vi "Button_handling1.vi"(7 "connect":bool, 10 "Z_Source":T2=enum."local disabled", 11 "Z_HSwitch":bool) -> (1 "Z_HSwitch_out":T1, 2 "Z1 ind":u8(ring), 3 "Write Enable":bool)   [LabVIEW 2019]
uses:
  Y_source.ctl
  Button state1.ctl
  Trigers/D^.vi
  Logik/fronts.vi
  Timer Delay/Timers.lvlib
  Counter/Counter.lvlib
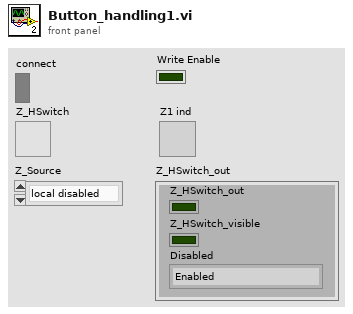
[diagram p1: front panel]
types:
  T1 = cluster{"Z_HSwitch_out":bool, "Z_HSwitch_visible":bool, "Disabled":enum8{"Enabled", "Disabled", "Disabled and Grayed Out"}}
  T2 = typedef "Y_source.ctl" = enum8{"initialize", "local disabled", "local hand", "hand", "auto", "dist"}
  T3 = enum8{"Enabled", "Disabled", "Disabled and Grayed Out"}
  T4 = typedef "Button state1.ctl" = enum16{"set init", "init", "set not connect", "not connect", "set local disabled", "local disabled", "set local hand", "local hand", "set hand", "hand", "set auto", "auto", "set dist", "dist"}
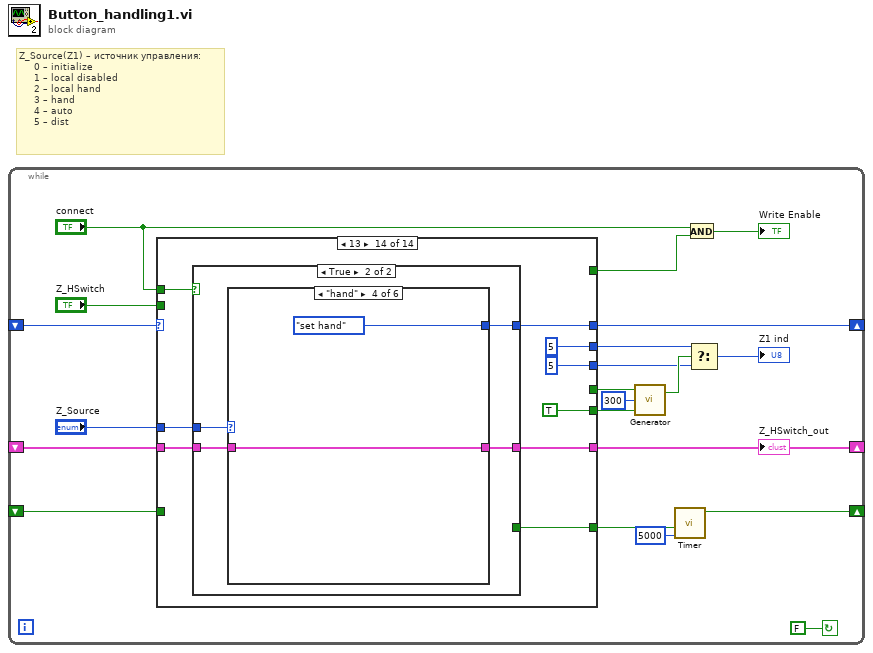
[diagram p0: block diagram]
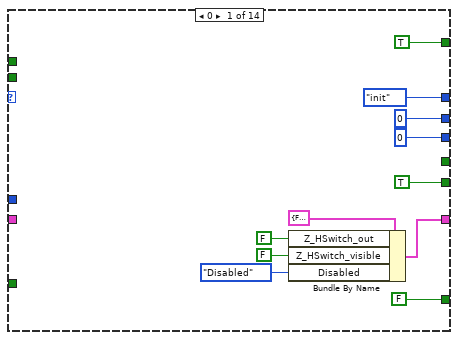
[diagram p2: hidden frame]
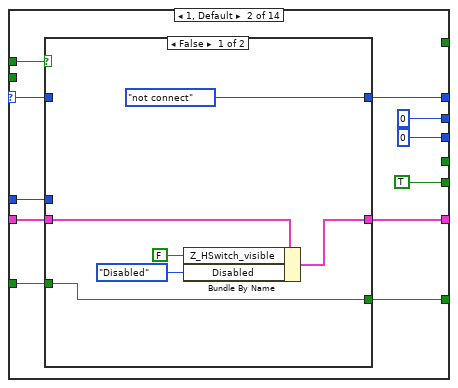
[diagram p3: hidden frame]
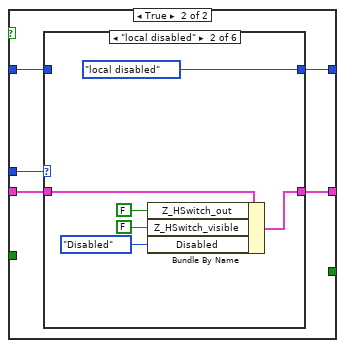
[diagram p4: hidden frame]
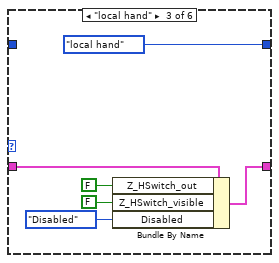
[diagram p6: hidden frame]
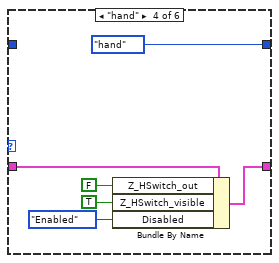
[diagram p7: hidden frame]
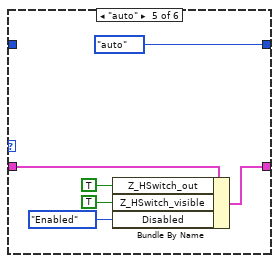
[diagram p8: hidden frame]
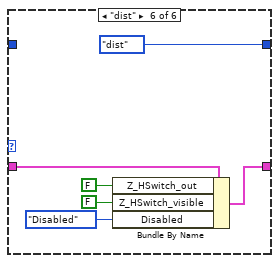
[diagram p9: hidden frame]
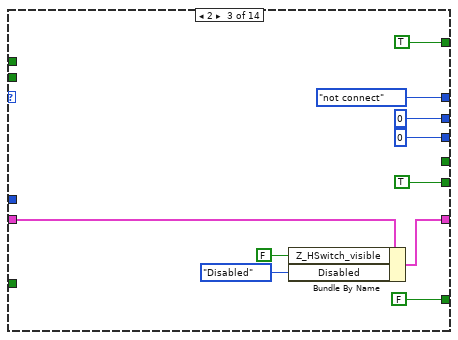
[diagram p10: hidden frame]
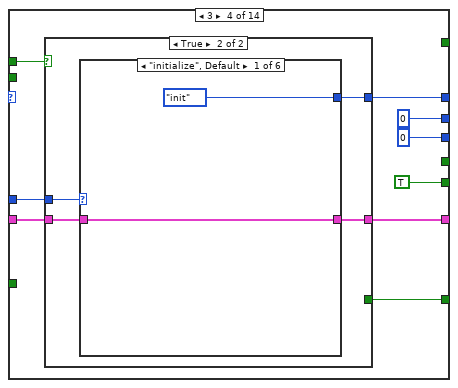
[diagram p11: hidden frame]
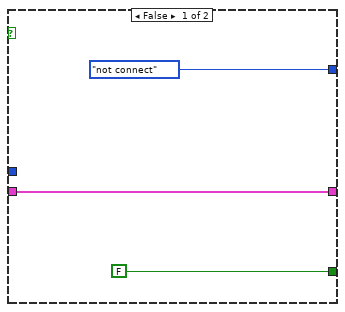
[diagram p12: hidden frame]
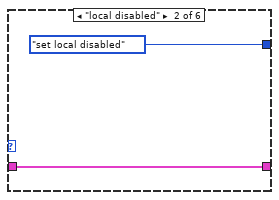
[diagram p13: hidden frame]
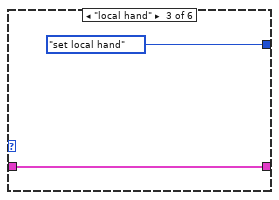
[diagram p14: hidden frame]
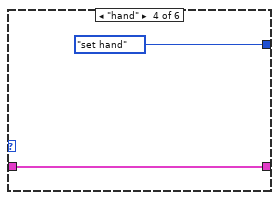
[diagram p15: hidden frame]
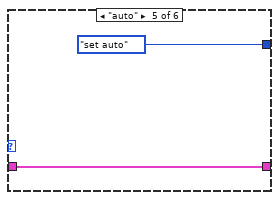
[diagram p16: hidden frame]
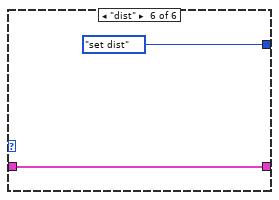
[diagram p17: hidden frame]
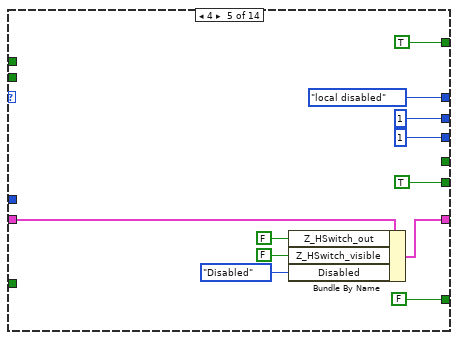
[diagram p18: hidden frame]
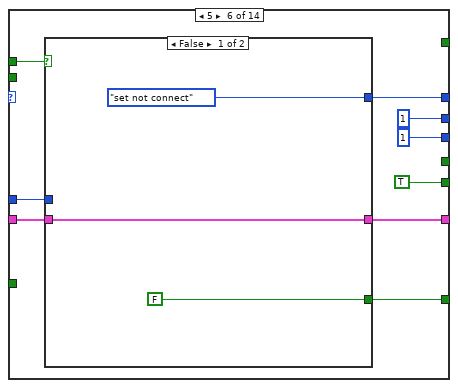
[diagram p19: hidden frame]
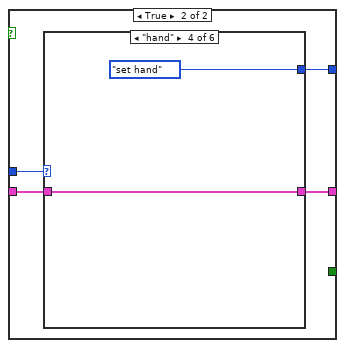
[diagram p20: hidden frame]
diagram:
  # "Z_Source(Z1) – источник управления:\n     0 – initialize\n     1 – local disabled\n     2 – local hand\n     3 – hand\n     4 – аuto\n     5 – dist"
  n1 = while {
    shift-right: [w21] -> _
    shift-left: _ -> [w7]
    shift-right: [w8] -> _
    shift-left: _ -> [w20]
    shift-right: [w4] -> _
    shift-left: _ -> [w9]
    stop <- FALSE continue-if-true
    n2 = case shown="13" w7 {
      selector: w7 -> [_ w33 _ _ _ _ _ _ _ _ _ _ _ _]
      tunnel: "connect" -> [_ w42 _ w104 _ w141 _ w180 w211 w255 w307 w351 _ w412]
      tunnel: "Z_HSwitch" -> [_ _ _ _ _ _ _ _ _ w257 _ w353 _ _]
      tunnel: [Button_state1."init" ("f 3") w43 Button_state1."not connect" ("f 3") w105 Button_state1."local disabled" ("f 3") w136 Button_state1."local hand" ("f 3") w179 w212 w256 w308 w352 Button_state1."dist" ("f 3") w413] -> w21
      tunnel: "Z_Source" -> [_ w41 _ w103 _ w138 _ w177 w210 w254 w306 w350 _ w411]
      tunnel: w20 -> [_ w34 _ _ _ _ _ _ w205 _ w301 _ _ _]
      tunnel: [FALSE ("Z_ASwitch") w40 FALSE ("Z_ASwitch") w102 FALSE ("Z_ASwitch") w137 FALSE ("Z_ASwitch") w175 w209 w253 w305 w349 FALSE ("Z_ASwitch") w408] -> w19
      tunnel: [u8 0 ("Z1 ind") u8 0 ("Z1 ind") u8 0 ("Z1 ind") u8 0 ("Z1 ind") u8 1 ("Z1 ind") u8 1 ("Z1 ind") u8 2 ("Z1 ind") u8 2 ("Z1 ind") u8 3 ("Z1 ind") u8 4 ("Z1 ind") u8 4 ("Z1 ind") u8 4 ("Z1 ind") u8 5 ("Z1 ind") u8 5 ("Z1 ind")] -> w12
      tunnel: [_ _ _ _ _ _ _ _ TRUE ("Z_ASwitch") w250 TRUE ("Z_ASwitch") w345 _ _] -> w17
      tunnel: [u8 0 ("Z1 ind") u8 0 ("Z1 ind") u8 0 ("Z1 ind") u8 0 ("Z1 ind") u8 1 ("Z1 ind") u8 1 ("Z1 ind") u8 2 ("Z1 ind") u8 2 ("Z1 ind") u8 4 ("Z1 ind") u8 3 ("Z1 ind") u8 3 ("Z1 ind") u8 4 ("Z1 ind") u8 5 ("Z1 ind") u8 5 ("Z1 ind")] -> w16
      tunnel: [TRUE ("Z_ASwitch") TRUE ("Z_ASwitch") TRUE ("Z_ASwitch") TRUE ("Z_ASwitch") TRUE ("Z_ASwitch") TRUE ("Z_ASwitch") TRUE ("Z_ASwitch") TRUE ("Z_ASwitch") _ w249 _ w346 TRUE ("Z_ASwitch") TRUE ("Z_ASwitch")] -> w15
      tunnel: [TRUE ("Z_ASwitch") _ TRUE ("Z_ASwitch") _ TRUE ("Z_ASwitch") _ TRUE ("Z_ASwitch") _ _ w246 _ w342 TRUE ("Z_ASwitch") _] -> w11
      tunnel: [w23 w36 w87 w98 w125 w140 w164 w178 w204 w248 w300 w344 w397 w409] -> w4
      tunnel: w9 -> [_ w35 w88 w97 w126 w139 w165 w176 w203 w247 w299 w343 w398 w410]
      frame 0 {
        # "local hand"
        n3 = Bundle By Name(cluster=T1 {"Z_HSwitch_out"=FALSE, "Z_HSwitch_visible"=FALSE, "Disabled"=enum."Enabled"} ("Z_HSwitch_out"), "Z_HSwitch_out"=FALSE ("Z_ASwitch"), "Z_HSwitch_visible"=FALSE ("Z_ASwitch"), "Disabled"=T3."Disabled") -> (w23:T1)
      }
      frame 1, Default {
        # "local hand"
        n4 = case shown="False" w42 {
          tunnel: [Button_state1."not connect" ("f 3") w54] -> w43
          tunnel: w41 -> [_ w53]
          tunnel: [w48 _] -> w40
          tunnel: [w44 w52] -> w36
          tunnel: w35 -> [w45 w51]
          tunnel: w34 -> [w48 _]
          tunnel: w33 -> [_ w50]
          frame False {
            # "not connect"
            n5 = Bundle By Name(cluster=w45, "Z_HSwitch_visible"=FALSE ("Z_ASwitch"), "Disabled"=T3."Disabled") -> (w44:T1)
          }
          frame True {
            # "not connect"
            n6 = case shown="\"local disabled\"" w53 {
              tunnel: [w55 Button_state1."local disabled" ("f 3") Button_state1."local hand" ("f 3") Button_state1."hand" ("f 3") Button_state1."auto" ("f 3") Button_state1."dist" ("f 3")] -> w54
              tunnel: [w56 w57 w63 w69 w75 w81] -> w52
              tunnel: w51 -> [w56 w58 w64 w70 w76 w82]
              tunnel: w50 -> [w55 _ _ _ _ _]
              frame "initialize", Default {
              }
              frame "local disabled" {
                n7 = Bundle By Name(cluster=w58, "Z_HSwitch_out"=FALSE ("Z_ASwitch"), "Z_HSwitch_visible"=FALSE ("Z_ASwitch"), "Disabled"=T3."Disabled") -> (w57:T1)
              }
              frame "local hand" {
                n8 = Bundle By Name(cluster=w64, "Z_HSwitch_out"=FALSE ("Z_ASwitch"), "Z_HSwitch_visible"=FALSE ("Z_ASwitch"), "Disabled"=T3."Disabled") -> (w63:T1)
              }
              frame "hand" {
                n9 = Bundle By Name(cluster=w70, "Z_HSwitch_out"=FALSE ("Z_ASwitch"), "Z_HSwitch_visible"=TRUE ("Z_ASwitch"), "Disabled"=T3."Enabled") -> (w69:T1)
              }
              frame "auto" {
                n10 = Bundle By Name(cluster=w76, "Z_HSwitch_out"=TRUE ("Z_ASwitch"), "Z_HSwitch_visible"=TRUE ("Z_ASwitch"), "Disabled"=T3."Enabled") -> (w75:T1)
              }
              frame "dist" {
                n11 = Bundle By Name(cluster=w82, "Z_HSwitch_out"=FALSE ("Z_ASwitch"), "Z_HSwitch_visible"=FALSE ("Z_ASwitch"), "Disabled"=T3."Disabled") -> (w81:T1)
              }
            }
          }
        }
      }
      frame 2 {
        # "local hand"
        n12 = Bundle By Name(cluster=w88, "Z_HSwitch_visible"=FALSE ("Z_ASwitch"), "Disabled"=T3."Disabled") -> (w87:T1)
      }
      frame 3 {
        # "local hand"
        n13 = case shown="True" w104 {
          tunnel: [Button_state1."not connect" ("f 3") w112] -> w105
          tunnel: w103 -> [_ w111]
          tunnel: [FALSE ("Z_ASwitch") _] -> w102
          tunnel: [w106 w110] -> w98
          tunnel: w97 -> [w106 w109]
          frame False {
            # "not connect"
          }
          frame True {
            # "not connect"
            n14 = case shown="\"initialize\", Default" w111 {
              tunnel: [Button_state1."init" ("f 3") Button_state1."set local disabled" ("f 3") Button_state1."set local hand" ("f 3") Button_state1."set hand" ("f 3") Button_state1."set auto" ("f 3") Button_state1."set dist" ("f 3")] -> w112
              tunnel: [w113 w115 w117 w119 w121 w123] -> w110
              tunnel: w109 -> [w113 w115 w117 w119 w121 w123]
              frame "initialize", Default {
              }
              frame "local disabled" {
              }
              frame "local hand" {
              }
              frame "hand" {
              }
              frame "auto" {
              }
              frame "dist" {
              }
            }
          }
        }
      }
      frame 4 {
        # "local hand"
        n15 = Bundle By Name(cluster=w126, "Z_HSwitch_out"=FALSE ("Z_ASwitch"), "Z_HSwitch_visible"=FALSE ("Z_ASwitch"), "Disabled"=T3."Disabled") -> (w125:T1)
      }
      frame 5 {
        # "local hand"
        n16 = case shown="False" w141 {
          tunnel: [Button_state1."set not connect" ("f 3") w151] -> w136
          tunnel: w138 -> [_ w150]
          tunnel: [FALSE ("Z_ASwitch") _] -> w137
          tunnel: [w145 w149] -> w140
          tunnel: w139 -> [w145 w148]
          frame False {
            # "not connect"
          }
          frame True {
            # "not connect"
            n17 = case shown="\"hand\"" w150 {
              tunnel: [Button_state1."init" ("f 3") Button_state1."set local disabled" ("f 3") Button_state1."set local hand" ("f 3") Button_state1."set hand" ("f 3") Button_state1."set auto" ("f 3") Button_state1."set dist" ("f 3")] -> w151
              tunnel: [w152 w154 w156 w158 w160 w162] -> w149
              tunnel: w148 -> [w152 w154 w156 w158 w160 w162]
              frame "initialize", Default {
              }
              frame "local disabled" {
              }
              frame "local hand" {
              }
              frame "hand" {
              }
              frame "auto" {
              }
              frame "dist" {
              }
            }
          }
        }
      }
      frame 6 {
        # "local hand"
        n18 = Bundle By Name(cluster=w165, "Z_HSwitch_out"=FALSE ("Z_ASwitch"), "Z_HSwitch_visible"=FALSE ("Z_ASwitch"), "Disabled"=T3."Disabled") -> (w164:T1)
      }
      frame 7 {
        # "local hand"
        n19 = case shown="True" w180 {
          tunnel: [Button_state1."set not connect" ("f 3") w190] -> w179
          tunnel: w177 -> [_ w189]
          tunnel: [FALSE ("Z_ASwitch") _] -> w175
          tunnel: [w184 w188] -> w178
          tunnel: w176 -> [w184 w187]
          frame False {
            # "not connect"
          }
          frame True {
            # "not connect"
            n20 = case shown="\"hand\"" w189 {
              tunnel: [Button_state1."init" ("f 3") Button_state1."set local disabled" ("f 3") Button_state1."set local hand" ("f 3") Button_state1."set hand" ("f 3") Button_state1."set auto" ("f 3") Button_state1."set dist" ("f 3")] -> w190
              tunnel: [w191 w193 w195 w197 w199 w201] -> w188
              tunnel: w187 -> [w191 w193 w195 w197 w199 w201]
              frame "initialize", Default {
              }
              frame "local disabled" {
              }
              frame "local hand" {
              }
              frame "hand" {
              }
              frame "auto" {
              }
              frame "dist" {
              }
            }
          }
        }
      }
      frame 8 {
        # "local hand"
        n21 = case shown="True" w211 {
          tunnel: [Button_state1."set not connect" ("f 3") w220] -> w212
          tunnel: w210 -> [_ w219]
          tunnel: [FALSE ("Z_ASwitch") _] -> w209
          tunnel: w205 -> [_ w218]
          tunnel: [w213 w217] -> w204
          tunnel: w203 -> [w213 w216]
          frame False {
            # "not connect"
          }
          frame True {
            # "not connect"
            n22 = case shown="\"hand\"" w219 {
              tunnel: [Button_state1."init" ("f 3") Button_state1."set local disabled" ("f 3") Button_state1."set local hand" ("f 3") Button_state1."hand" ("f 3") w237 Button_state1."set dist" ("f 3")] -> w220
              tunnel: w218 -> [_ _ _ _ w232 _]
              tunnel: [w221 w223 w225 w227 w234 w244] -> w217
              tunnel: w216 -> [w221 w223 w225 w228 w233 w244]
              frame "initialize", Default {
              }
              frame "local disabled" {
              }
              frame "local hand" {
              }
              frame "hand" {
                n23 = Bundle By Name(cluster=w228, "Z_HSwitch_visible"=TRUE ("Z_ASwitch"), "Disabled"=T3."Enabled") -> (w227:T1)
              }
              frame "auto" {
                n24 = case shown="True" w232 {
                  tunnel: [w238 w239] -> w234
                  tunnel: w233 -> [w238 w240]
                  frame False {
                  }
                  frame True {
                    n25 = Bundle By Name(cluster=w240, "Z_HSwitch_out"=TRUE ("Z_ASwitch"), "Z_HSwitch_visible"=TRUE ("Z_ASwitch"), "Disabled"=T3."Enabled") -> (w239:T1)
                  }
                }
                n26 = Select(t=Button_state1."auto" ("f 3"), s=w232, f=Button_state1."set hand" ("f 3")) -> (s? t:f=w237:T4)
              }
              frame "dist" {
              }
            }
          }
        }
      }
      frame 9 {
        # "local hand"
        n27 = case shown="True" w255 {
          tunnel: w257 -> [_ w267]
          tunnel: [Button_state1."set not connect" ("f 3") w269] -> w256
          tunnel: w254 -> [_ w268]
          tunnel: [_ w266] -> w253
          tunnel: [_ w265] -> w250
          tunnel: [TRUE ("Z_ASwitch") w264] -> w249
          tunnel: [w258 w263] -> w248
          tunnel: w247 -> [w258 w262]
          tunnel: [_ w261] -> w246
          frame False {
            # "not connect"
          }
          frame True {
            # "not connect"
            n28 = case shown="\"hand\"" w268 {
              tunnel: [Button_state1."init" ("f 3") Button_state1."set local disabled" ("f 3") Button_state1."set local hand" ("f 3") w284 Button_state1."set auto" ("f 3") Button_state1."set dist" ("f 3")] -> w269
              tunnel: w267 -> [_ _ _ w279 _ _]
              tunnel: [_ _ _ w280 _ _] -> w266
              tunnel: [_ _ _ w279 _ _] -> w265
              tunnel: [TRUE ("Z_ASwitch") TRUE ("Z_ASwitch") TRUE ("Z_ASwitch") _ TRUE ("Z_ASwitch") TRUE ("Z_ASwitch")] -> w264
              tunnel: [w270 w273 w276 w282 w293 w296] -> w263
              tunnel: w262 -> [w270 w273 w276 w281 w293 w296]
              tunnel: [_ _ _ w279 _ _] -> w261
              frame "initialize", Default {
              }
              frame "local disabled" {
              }
              frame "local hand" {
              }
              frame "hand" {
                n29 = case shown="True" w279 {
                  tunnel: [w286 w288] -> w282
                  tunnel: w281 -> [w286 w289]
                  tunnel: [_ TRUE ("Z_ASwitch")] -> w280
                  frame False {
                  }
                  frame True {
                    n30 = Bundle By Name(cluster=w289, "Z_HSwitch_out"=TRUE ("Z_ASwitch"), "Z_HSwitch_visible"=FALSE ("Z_ASwitch"), "Disabled"=T3."Disabled") -> (w288:T1)
                  }
                }
                n31 = Select(t=Button_state1."set auto" ("f 3"), s=w279, f=Button_state1."hand" ("f 3")) -> (s? t:f=w284:T4)
              }
              frame "auto" {
              }
              frame "dist" {
              }
            }
          }
        }
      }
      frame 10 {
        # "local hand"
        n32 = case shown="True" w307 {
          tunnel: [Button_state1."set not connect" ("f 3") w316] -> w308
          tunnel: w306 -> [_ w315]
          tunnel: [FALSE ("Z_ASwitch") _] -> w305
          tunnel: w301 -> [_ w314]
          tunnel: [w309 w313] -> w300
          tunnel: w299 -> [w309 w312]
          frame False {
            # "not connect"
          }
          frame True {
            # "not connect"
            n33 = case shown="\"auto\"" w315 {
              tunnel: [Button_state1."init" ("f 3") Button_state1."set local disabled" ("f 3") Button_state1."set local hand" ("f 3") w328 Button_state1."auto" ("f 3") Button_state1."set dist" ("f 3")] -> w316
              tunnel: w314 -> [_ _ _ w323 _ _]
              tunnel: [w317 w319 w321 w325 w335 w340] -> w313
              tunnel: w312 -> [w317 w319 w321 w324 w336 w340]
              frame "initialize", Default {
              }
              frame "local disabled" {
              }
              frame "local hand" {
              }
              frame "hand" {
                n34 = case shown="True" w323 {
                  tunnel: [w329 w331] -> w325
                  tunnel: w324 -> [w329 w330]
                  frame False {
                  }
                  frame True {
                    n35 = Bundle By Name(cluster=w330, "Z_HSwitch_out"=FALSE ("Z_ASwitch"), "Z_HSwitch_visible"=TRUE ("Z_ASwitch"), "Disabled"=T3."Enabled") -> (w331:T1)
                  }
                }
                n36 = Select(t=Button_state1."hand" ("f 3"), s=w323, f=Button_state1."set auto" ("f 3")) -> (s? t:f=w328:T4)
              }
              frame "auto" {
                n37 = Bundle By Name(cluster=w336, "Z_HSwitch_visible"=TRUE ("Z_ASwitch"), "Disabled"=T3."Enabled") -> (w335:T1)
              }
              frame "dist" {
              }
            }
          }
        }
      }
      frame 11 {
        # "local hand"
        n38 = case shown="True" w351 {
          tunnel: w353 -> [_ w364]
          tunnel: [Button_state1."set not connect" ("f 3") w366] -> w352
          tunnel: w350 -> [_ w365]
          tunnel: [FALSE ("Z_ASwitch") w363] -> w349
          tunnel: [TRUE ("Z_ASwitch") w362] -> w346
          tunnel: [_ w361] -> w345
          tunnel: [w354 w360] -> w344
          tunnel: w343 -> [w354 w359]
          tunnel: [_ w358] -> w342
          frame False {
            # "not connect"
          }
          frame True {
            # "not connect"
            n39 = case shown="\"auto\"" w365 {
              tunnel: [Button_state1."init" ("f 3") Button_state1."set local disabled" ("f 3") Button_state1."set local hand" ("f 3") Button_state1."set hand" ("f 3") w385 Button_state1."set dist" ("f 3")] -> w366
              tunnel: w364 -> [_ _ _ _ w383 _]
              tunnel: [_ _ _ _ w380 _] -> w363
              tunnel: [TRUE ("Z_ASwitch") TRUE ("Z_ASwitch") TRUE ("Z_ASwitch") TRUE ("Z_ASwitch") _ TRUE ("Z_ASwitch")] -> w362
              tunnel: [_ _ _ _ w379 _] -> w361
              tunnel: [w367 w370 w373 w376 w382 w394] -> w360
              tunnel: w359 -> [w367 w370 w373 w376 w381 w394]
              tunnel: [_ _ _ _ w379 _] -> w358
              frame "initialize", Default {
              }
              frame "local disabled" {
              }
              frame "local hand" {
              }
              frame "hand" {
              }
              frame "auto" {
                n40 = case shown="False" w383 {
                  tunnel: [w387 w389] -> w382
                  tunnel: w381 -> [w387 w390]
                  tunnel: [_ TRUE ("Z_ASwitch")] -> w380
                  frame True {
                  }
                  frame False {
                    n41 = Bundle By Name(cluster=w390, "Z_HSwitch_out"=FALSE ("Z_ASwitch"), "Z_HSwitch_visible"=FALSE ("Z_ASwitch"), "Disabled"=T3."Disabled") -> (w389:T1)
                  }
                }
                n42 = Select(t=Button_state1."auto" ("f 3"), s=w383, f=Button_state1."set hand" ("f 3")) -> (s? t:f=w385:T4)
                n43 = Not(x=w383) -> (.not. x?=w379:bool)
              }
              frame "dist" {
              }
            }
          }
        }
      }
      frame 12 {
        # "local hand"
        n44 = Bundle By Name(cluster=w398, "Z_HSwitch_out"=FALSE ("Z_ASwitch"), "Z_HSwitch_visible"=FALSE ("Z_ASwitch"), "Disabled"=T3."Disabled") -> (w397:T1)
      }
      frame 13 {
        # "local hand"
        n45 = case shown="True" w412 {
          tunnel: [Button_state1."set not connect" ("f 3") w423] -> w413
          tunnel: w411 -> [_ w422]
          tunnel: [FALSE ("Z_ASwitch") _] -> w408
          tunnel: [w417 w421] -> w409
          tunnel: w410 -> [w417 w420]
          frame False {
            # "not connect"
          }
          frame True {
            # "not connect"
            n46 = case shown="\"hand\"" w422 {
              tunnel: [Button_state1."init" ("f 3") Button_state1."set local disabled" ("f 3") Button_state1."set local hand" ("f 3") Button_state1."set hand" ("f 3") Button_state1."set auto" ("f 3") Button_state1."set dist" ("f 3")] -> w423
              tunnel: [w424 w426 w428 w430 w432 w434] -> w421
              tunnel: w420 -> [w424 w426 w428 w430 w432 w434]
              frame "initialize", Default {
              }
              frame "local disabled" {
              }
              frame "local hand" {
              }
              frame "hand" {
              }
              frame "auto" {
              }
              frame "dist" {
              }
            }
          }
        }
      }
    }
    "Z_HSwitch_out" <- w4
    n47 = call "Generator.vi"("R"=w15, "T ms (500)"=300, "ON (F)"=w17) -> ("Q"=w18:bool)  [unwired: 1 in]
    n48 = call "Timer.vi"("ms"=5000, "Load (F)"=w19) -> ("End"=w8:bool)  [unwired: 7 in, 1 out]
    n49 = And(x="connect", y=w11) -> (x .and. y?=→"Write Enable":bool)
    n50 = Select(t=w12, s=w18, f=w16) -> (s? t:f=→"Z1 ind":u8)
  }
